vi "Reset.vi"(8 "error in (no error)":errorcluster, 11 "U1252 in":refnum<class "U1252.lvclass">) -> (0 "error out":errorcluster, 3 "U1252 out":refnum<class "U1252.lvclass">)   [LabVIEW 2015, in "U1252.lvclass"]
uses:
  U1252.lvclass
  <instrlib>/U1250 Series Multimeter Device Driver/U1250 Series Digital Multimeter.lvlib
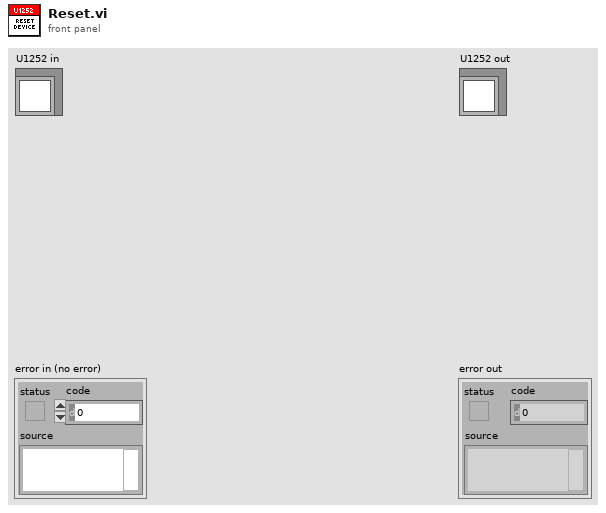
[diagram p1: front panel]
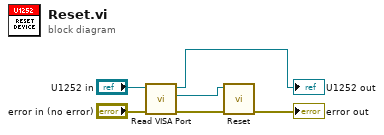
[diagram p0: block diagram]
diagram:
  n1 = call-dynamic "Read VISA Port.vi"("error in (no error)"="error in (no error)", "Device in"="U1252 in") -> ("error out"=w2:errorcluster, "VISA Port"=w3:refnum<visa-resource-name>, "Device out"=→"U1252 out":refnum<class "U1252.lvclass">)  [unwired: 7 in]
  n2 = call <instrlib>:"Reset.vi"("error in (no error)"=w2, "VISA resource name"=w3) -> ("error out"=→"error out":errorcluster)  [unwired: 8 in, 1 out]
